vi "RunIconEditorvi.vi"(7 "CtlRef":refnum<vi>, 8 "error in (no error)":errorcluster, 11 "VI Refnum in":refnum<vi>) -> (0 "error out":errorcluster)   [LabVIEW 2014, in "GCMIconEditor.lvlib" / "GCMIconEditor.lvclass"]
uses:
  GCMIconEditor.lvclass
  <vilib>/LabVIEW Icon API/LabVIEW Icon API.lvlib
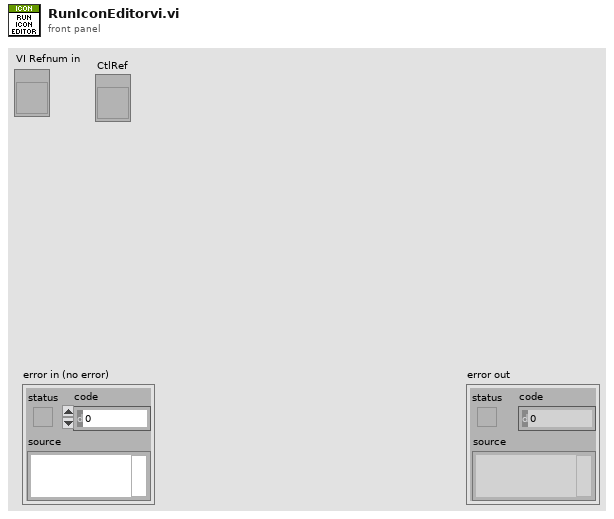
[diagram p1: front panel]
types:
  T1 = typedef "imagedata.ctl" = cluster{"image type":i32, "image depth":i32, "image":u8[], "mask":u8[], "colors":u32[], "Rectangle":cluster{"left":i16, "top":i16, "right":i16, "bottom":i16}}
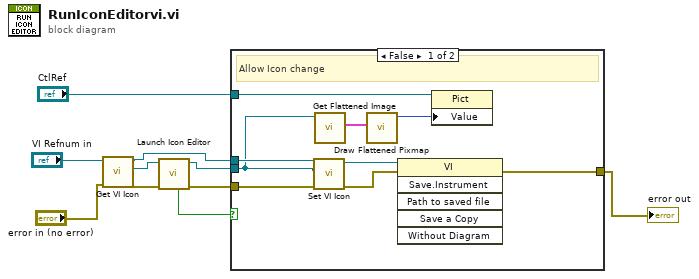
[diagram p0: block diagram]
diagram:
  n1 = call <vilib>:"Get VI Icon.vi"("error in (no error)"="error in (no error)", "VI Refnum in"="VI Refnum in") -> ("error out"=w5:errorcluster, "Icon"=w6:refnum<class "Icon.lvclass">, "VI Refnum out"=w7:refnum<vi>)  [unwired: 7 in]
  n2 = call <vilib>:"Launch Icon Editor.vi"("error in (no error)"=w5, "Icon in"=w6) -> ("error out"=w10:errorcluster, "Icon out"=w9:refnum<class "Icon.lvclass">, "Canceled?"=w8:bool)  [unwired: 7 in]
  n3 = case shown="False" w8 {
    tunnel: w7 -> [w16 _]
    tunnel: w10 -> [w15 w20]
    tunnel: w9 -> [w14 _]
    tunnel: [w13 w20] -> w3
    tunnel: "CtlRef" -> [w12 _]
    frame False {
      # "Allow Icon change"
      n4 = call <vilib>:"Set VI Icon.vi"("error in (no error)"=w15, "Icon"=w14, "VI Refnum in"=w16) -> ("error out"=w18:errorcluster, "VI Refnum out"=w17:refnum<vi>)  [unwired: 7 in]
      n5 = call <vilib>:"Get Flattened Image.vi"("lv_icon.lvlib:Icon.lvclass in"=w14) -> ("Color Image"=w19:T1)  [unwired: 7 in, 3 out]
      n6 = call <vilib>:"Draw Flattened Pixmap.vi"("image data"=w19) -> ("new picture"=w11:picture)  [unwired: 8 in]
      n7 = invoke class="VI" method="Save.Instrument"(reference=w17, error in=w18) -> (error out=w13:errorcluster)  [unwired: 4 in, 5 out]
      n8 = property class="Pict"(reference=w12, "Value"=w11) -> ()  [unwired: 1 in, 2 out]
    }
    frame True {
      # "Cancel operation"
    }
  }
  "error out" <- w3
